vi "Address.vi"(11 "Address_input":string) -> (3 "Address":string)   [LabVIEW 2020]
uses:
  DLL_Address.dll
panel:
  out "*(type *) &x":i32 format="%.0x"
  out "error out":u16
  out "size":i32
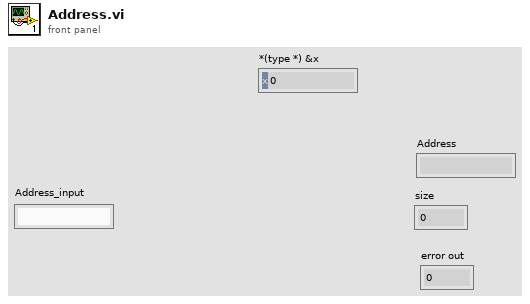
[diagram p1: front panel]
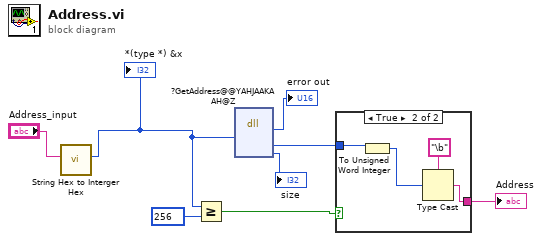
[diagram p0: block diagram]
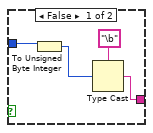
[diagram p2: hidden frame]
diagram:
  n1 = call "String Hex to Interger Hex.vi"("Hex Display Input"="Address_input") -> ("Integer Decimal Equivalent"=w1:i32)  [unwired: 10 in]
  "*(type *) &x" <- w1
  n2 = Greater Or Equal?(x=w1, y=256) -> (x >= y?=w5:bool)
  n3 = dll-call lib="E:/USB/KTC/Instrument/Electricity center/Electricity meter_DLMS/Subvi/DLL_Address.dll" fn="?GetAddress@@YAHJAAKAAH@Z"("value"=w1) -> ("error out"=→"error out":u16, "address"=w4:u32, "size"=→"size":i32)  [unwired: 6 in, 2 out]
  n4 = case shown="True" w5 {
    tunnel: w4 -> [w12 w16]
    tunnel: [w9 w13] -> w3
    frame False {
      n5 = To Unsigned Byte Integer(number=w12) -> (unsigned 8bit integer=w10:u8)
      n6 = Type Cast(type="\b", x=w10) -> (*(type *) &x=w9:string)
    }
    frame True {
      n7 = To Unsigned Word Integer(number=w16) -> (unsigned 16bit integer=w14:u16)
      n8 = Type Cast(type="\b", x=w14) -> (*(type *) &x=w13:string)
    }
  }
  "Address" <- w3
